vi "test_extended_depth.vi"() -> ()   [LabVIEW 2023]
uses:
  <vilib>/picture/picture.llb/Draw True-Color Pixmap.vi
panel:
  out "metadata":cluster{"width":u16, "height":u16}
  in  "media_index":u64=13
  in  "profile_index":sgl
  in  "source_index":sgl
  in  "group_index":sgl
  out "Depth (modified)":picture
  in  "host":string="192.168.1.7"
  in  "path in":path=path "C:/Users/jcds/Documents/GitHub/hl2ss/extensions/client_labview/hl2ss_labview/hl2ss_ulm.dll"
  in  "stop":bool
  out "pose":sgl[][](array[numeric])
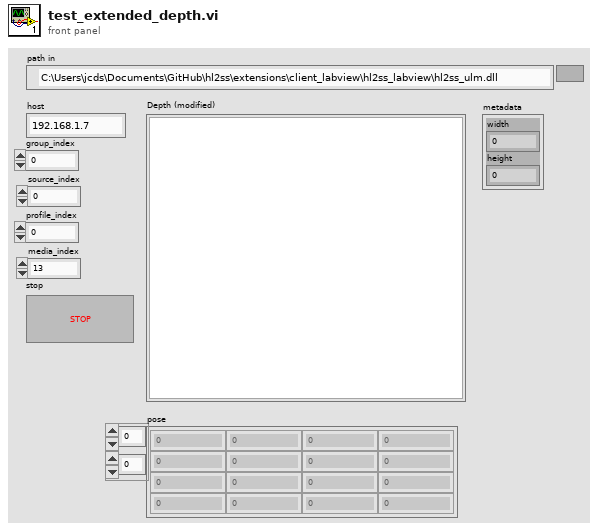
[diagram p1: front panel]
types:
  T1 = cluster{"enable_mrc":u8, "hologram_composition":u8, "recording_indicator":u8, "video_stabilization":u8, "blank_protected":u8, "show_mesh":u8, "shared":u8, "_reserved_0":u8, "global_opacity":sgl, "output_width":sgl, "output_height":sgl, "video_stabilization_length":u32, "hologram_perspective":u32, "_reserved_1":u32}
  T2 = cluster{"chunk":u64, "media_index":u64, "stride_mask":u64, "mode":u8, "divisor":u8, "profile_z":u8, "_reserved_0":u8, "_reserved_1":u8, "_reserved_2":u8, "_reserved_3":u8, "_reserved_4":u8}
  T3 = cluster{"frame_stamp":i64, "timestamp":u64, "payload_size":u32, "status":i32, "payload":u64, "pose":u64}
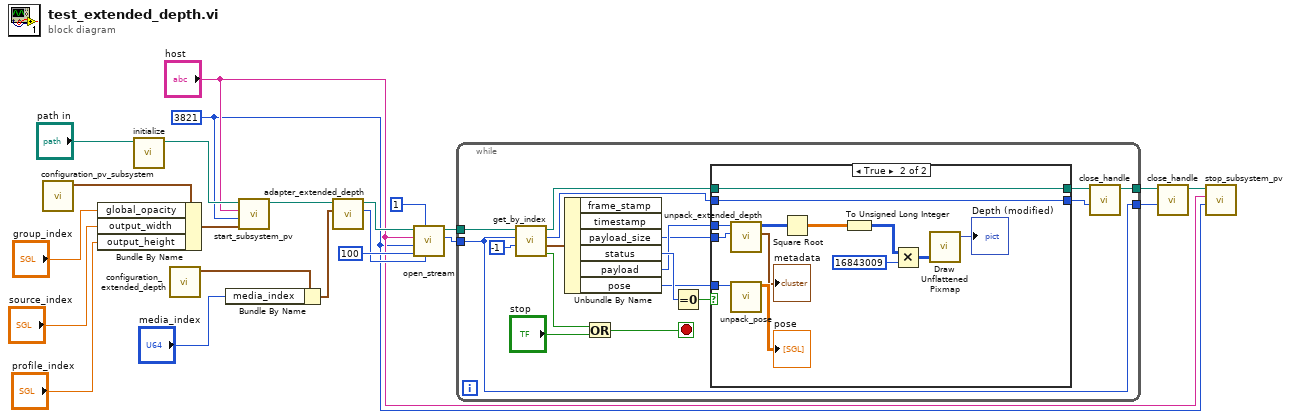
[diagram p0: block diagram]
diagram:
  w9 = u16 3821 ("port")
  n1 = call "configuration_pv_subsystem.vi"() -> ("configuration_pv_subsystem"=w8:T1)  [unwired: 11 in]
  n2 = Bundle By Name(cluster=w8, "global_opacity"="group_index", "output_width"="source_index", "output_height"="profile_index") -> (w4:T1)
  n3 = call "initialize.vi"("path in"="path in") -> ("path out"=w12:path)  [unwired: 9 in, 1 out]
  n4 = call "configuration_extended_depth.vi"() -> ("configuration_extended_depth"=w3:T2)  [unwired: 11 in]
  n5 = Bundle By Name(cluster=w3, "media_index"="media_index") -> (w1:T2)
  n6 = call "start_subsystem_pv.vi"("configuration"=w4, "port"=w9, "host"="host", "path in"=w12) -> ("path out"=w11:path)  [unwired: 6 in, 1 out]
  n7 = call "adapter_extended_depth.vi"("configuration_extended_depth"=w1, "path in"=w11) -> ("configuration"=w15:u64, "path out"=w14:path)  [unwired: 8 in]
  n8 = call "open_stream.vi"("configuration"=w15, "decoded"=u8 1, "buffer_size"=u64 100, "port"=w9, "host"="host", "path in"=w14) -> ("handle"=w22:u64, "path out"=w21:path)  [unwired: 3 in, 1 out]
  n9 = while {
    tunnel: [w30] -> w18
    tunnel: w22 -> [w24]
    tunnel: w21 -> [w25]
    tunnel: [w24] -> w17
    stop <- w29 stop-if-true
    n10 = call "get_by_index.vi"("frame_stamp"=i64 -1, "stream_handle"=w24, "path in"=w25) -> ("error"=w28:bool, "packet"=w39:T3, "packet_handle"=w33:u64, "path out"=w32:path)  [unwired: 5 in]
    n11 = Unbundle By Name(w39) -> ("payload_size"=w23:u32, "status"=w38:i32, "payload"=w36:u64, "pose"=w35:u64)  [unwired: 2 out]
    n12 = Or(x=w28, y="stop") -> (x .or. y?=w29:bool)
    n13 = Equal To 0?(x=w38) -> (x = 0?=w37:bool)
    n14 = case shown="True" w37 {
      tunnel: w36 -> [_ w45]
      tunnel: w35 -> [_ w52]
      tunnel: [w40 w54] -> w34
      tunnel: w33 -> [w40 w54]
      tunnel: w32 -> [w41 w53]
      tunnel: [w41 w53] -> w31
      tunnel: w23 -> [_ w44]
      frame False {
      }
      frame True {
        n15 = call "unpack_extended_depth.vi"("payload_size"=w44, "payload"=w45) -> ("metadata"=→"metadata":cluster{"width":u16, "height":u16}, "image"=w43:u16[][])  [unwired: 5 in, 3 out]
        n16 = call "unpack_pose.vi"("pose"=w52) -> ("pose"=→"pose":sgl[][])  [unwired: 9 in, 1 out]
        n17 = Square Root(x=w43) -> (sqrt(x)=w50:dbl[][])
        n18 = To Unsigned Long Integer(number=w50) -> (unsigned 32bit integer=w49:u32[][])
        n19 = Multiply(x=w49, y=u32 16843009 ("frame_stamp")) -> (x*y=w47:u32[][])
        n20 = call-poly <vilib>:"Draw Unflattened Pixmap.vi"("data (RGB format)"=w47) -> ("new picture"=→"Depth (modified)":picture)  [unwired: 8 in]
      }
    }
    n21 = call "close_handle.vi"("handle"=w34, "path in"=w31) -> ("path out"=w30:path)  [unwired: 9 in]
  }
  n22 = call "close_handle.vi"("handle"=w17, "path in"=w18) -> ("path out"=w13:path)  [unwired: 9 in]
  n23 = call "stop_subsystem_pv.vi"("port"=w9, "host"="host", "path in"=w13) -> ()  [unwired: 7 in, 2 out]
